vi "fix class control labels.vi"(8 "error in":errorcluster, 10 "class to load":path, 11 "Application in":refnum<vi>) -> (0 "error out":errorcluster)   [LabVIEW 2013, in "TagBusProcessingPluginFeatureDecider.lvclass"]
uses:
  TagBusProcessingPluginFeatureDecider.lvclass
  <vilib>/Utility/traverseref.llb/TRef TravTarget.ctl
  <vilib>/Utility/traverseref.llb/VI Scripting - Traverse.lvlib
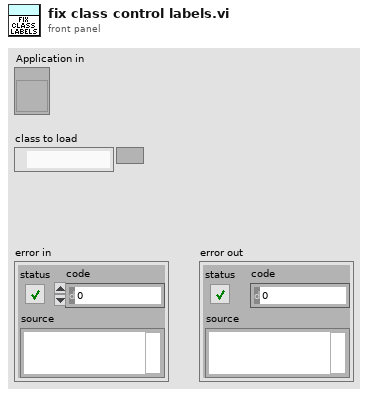
[diagram p1: front panel]
types:
  T1 = typedef "TRef TravTarget.ctl" = enum16{"FP", "BD", "Other"}
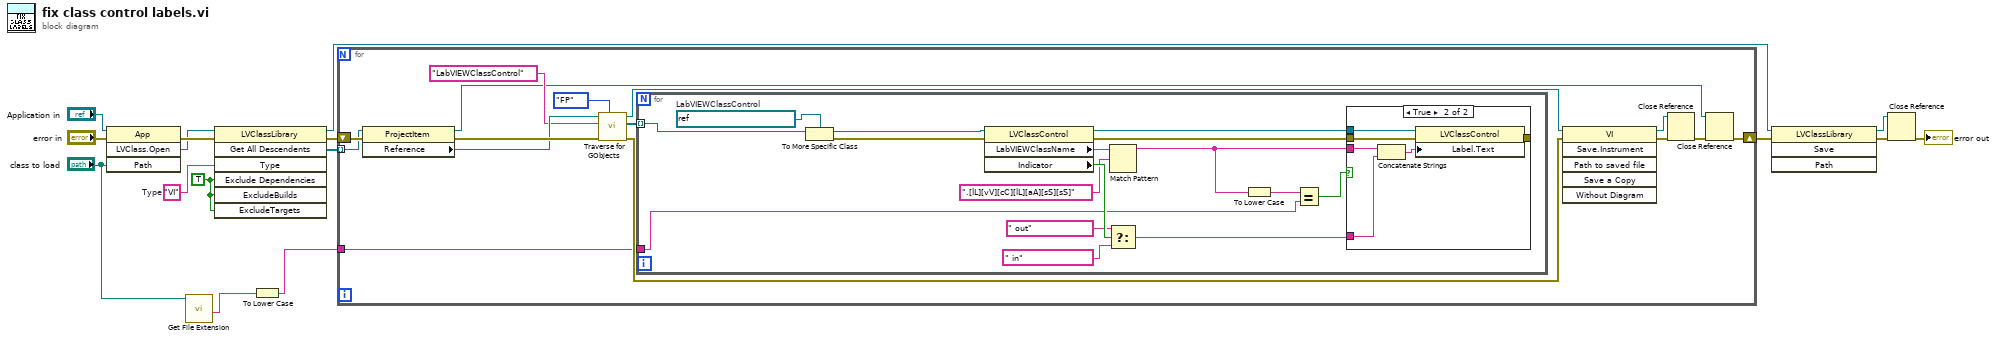
[diagram p0: block diagram]
diagram:
  w12 = TRUE
  w11 = "VI"  # Type
  n1 = invoke class="App" method="LVClass.Open"(reference="Application in", error in="error in", "Path"="class to load") -> (error out=w13:errorcluster, "LVClass.Open"=w10:refnum<vi>)  [unwired: 1 in, 2 out]
  n2 = call <vilib>:"Get File Extension.vi"("file"="class to load") -> ("filename without extension"=w2:string)  [unwired: 7 in, 3 out]
  n3 = invoke class="LVClassLibrary" method="Get All Descendents"(reference=w10, error in=w13, "Type"=w11, "Exclude Dependencies"=w12, "ExcludeBuilds"=w12, "ExcludeTargets"=w12) -> (reference out=w8:refnum<vi>, error out=w15:errorcluster, "All Descendents"=w14:refnum<vi>[])  [unwired: 1 in, 4 out]
  n4 = To Lower Case(string=w2) -> (all lower case string=w1:string)
  n5 = for {
    tunnel: w14 -> [w30] mode=indexing
    shift-right: [w22] -> w16
    shift-left: w15 -> [w31]
    tunnel: w1 -> [w17]
    n6 = property class="ProjectItem"(reference=w30, error in=w31) -> (reference out=w21:refnum<vi>, error out=w29:errorcluster, "Reference"=w28:refnum<vi>)
    n7 = call <vilib>:"Traverse for GObjects.vi"("Traverse Target"=TRef_TravTarget."FP", "error in (no error)"=w29, "Class Name"="LabVIEWClassControl", "VI Refnum"=w28) -> ("error out"=w18:errorcluster, "References"=w25:refnum<vi>[], "dup VI Refnum"=w24:refnum<vi>)  [unwired: 4 in, 1 out]
    n8 = for {
      tunnel: w25 -> [w46] mode=indexing
      tunnel: w17 -> [w34]
      w44 = refnum<vi> refnum  # LabVIEWClassControl
      n9 = To More Specific Class(target class=w44, reference=w46) -> (specific class reference=w45:refnum<vi>, error out=w47:errorcluster)  [unwired: 1 in]
      n10 = property class="LVClassControl"(reference=w45, error in=w47) -> (reference out=w43:refnum<vi>, error out=w42:errorcluster, "LabVIEWClassName"=w37:string, "Indicator"=w41:bool)
      n11 = Match Pattern(string=w37, regular expression=".[lL][vV][cC][lL][aA][sS][sS]") -> (before substring=w35:string)  [unwired: 1 in, 3 out]
      n12 = Select(t=" out", s=w41, f=" in") -> (s? t:f=w38:string)
      n13 = To Lower Case(string=w35) -> (all lower case string=w33:string)
      n14 = Equal?(x=w33, y=w34) -> (x = y?=w32:bool)
      n15 = case shown="True" w32 {
        tunnel: w43 -> [_ w53]
        tunnel: w42 -> [_ w52]
        tunnel: w38 -> [_ w50]
        tunnel: [_ w49] -> _
        tunnel: w35 -> [_ w48]
        frame False {
        }
        frame True {
          n16 = Concatenate Strings(w48, w50) -> (w51:string)
          n17 = property class="LVClassControl"(reference=w53, error in=w52, "Label.Text"=w51) -> (error out=w49:errorcluster)  [unwired: 1 out]
        }
      }
    }
    n18 = invoke class="VI" method="Save.Instrument"(reference=w24, error in=w18) -> (reference out=w19:refnum<vi>, error out=w20:errorcluster)  [unwired: 4 in, 4 out]
    n19 = Close Reference(reference=w19, error in (no error)=w20) -> (error out=w23:errorcluster)
    n20 = Close Reference(reference=w21, error in (no error)=w23) -> (error out=w22:errorcluster)
  }
  n21 = invoke class="LVClassLibrary" method="Save"(reference=w8, error in=w16) -> (reference out=w7:refnum<vi>, error out=w9:errorcluster)  [unwired: 2 in, 2 out]
  n22 = Close Reference(reference=w7, error in (no error)=w9) -> (error out=→"error out":errorcluster)
